vi "testDataPass_v2,0_vi0_host.vi"() -> ()   [LabVIEW 2014]
uses:
  <vilib>/WebDAVClient/Advanced/Put File.vi
  <vilib>/WebDAVClient/NI_WebDAV.lvlib
panel:
  out "Boolean":bool
  out "error out":errorcluster
  out "code":i32
  out "error out 2":errorcluster
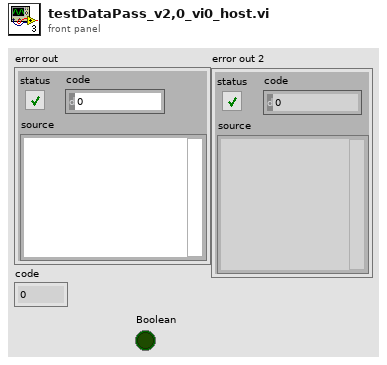
[diagram p1: front panel]
types:
  T1 = typedef "NI_WebDAV.lvlib/SessionHandle.ctl" = refnum<k1>
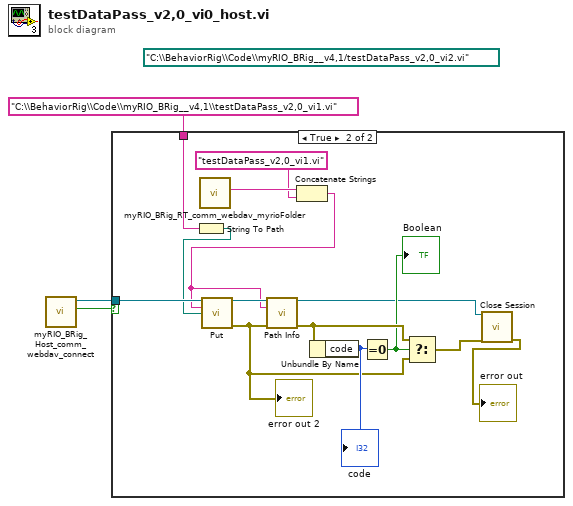
[diagram p0: block diagram]
diagram:
  (unwired) path "C:\\BehaviorRig\\Code\\myRIO_BRig__v4,1/testDataPass_v2,0_vi2.vi" ("vi path")
  n1 = call "myRIO_BRig_Host_comm_webdav_connect.vi"() -> ("output_Iconnected"=w3:bool, "output_hSession"=w1:T1)  [unwired: 9 in, 1 out]
  n2 = case shown="True" w3 {
    tunnel: "C:\\BehaviorRig\\Code\\myRIO_BRig__v4,1\\testDataPass_v2,0_vi1.vi" -> [_ w14]
    tunnel: w1 -> [_ w17]
    frame False {
    }
    frame True {
      n3 = String To Path(string=w14) -> (path=w13:path)
      n4 = call "myRIO_BRig_RT_comm_webdav_myrioFolder.vi"() -> ("output_myrioFolder"=w16:string)  [unwired: 11 in]
      n5 = Concatenate Strings(w16, "testDataPass_v2,0_vi1.vi" ("string")) -> (w10:string)
      n6 = call-poly <vilib>:"Put.vi"("session handle"=w17, "relative uri"=w10, "local file path"=w13) -> ("session handle out"=w12:T1, "error out"=w8:errorcluster)  [unwired: 10 in, 1 out]
      "error out 2" <- w8
      n7 = call <vilib>:"Path Info.vi"("session handle"=w12, "relative uri"=w10, "error in (no error)"=w8) -> ("session handle out"=w5:T1, "error out"=w9:errorcluster)  [unwired: 9 in, 2 out]
      n8 = Unbundle By Name(w9) -> ("code"=w11:i32)
      "code" <- w11
      n9 = Equal To 0?(x=w11) -> (x = 0?=w7:bool)
      "Boolean" <- w7
      n10 = Select(t=w9, s=w7, f=w8) -> (s? t:f=w4:errorcluster)
      n11 = call <vilib>:"Close Session.vi"("session handle"=w5, "error in (no error)"=w4) -> ("error out"=→"error out":errorcluster)  [unwired: 13 in]
    }
  }
